vi "Create Folder.vi"(8 "error in":errorcluster, 11 "Source Path":path) -> (0 "error out":errorcluster, 2 "Already Exists":bool, 3 "created path":path)   [LabVIEW 2014, in "Utilities.lvlib"]
uses:
  Utilities.lvlib
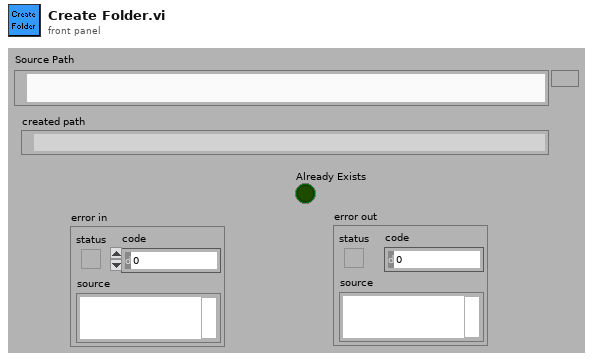
[diagram p1: front panel]
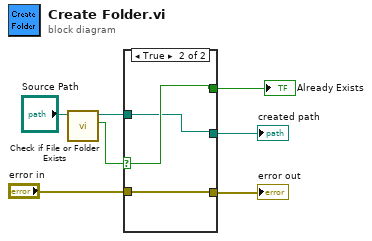
[diagram p0: block diagram]
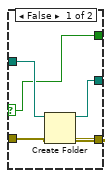
[diagram p2: hidden frame]
diagram:
  n1 = call <vilib>:"Check if File or Folder Exists.vi"("path"="Source Path") -> ("file or folder exists?"=w7:bool, "dup path"=w2:path)  [unwired: 8 in, 1 out]
  n2 = case shown="True" w7 {
    selector: w7 -> [w8 w15]
    tunnel: w2 -> [w11 w13]
    tunnel: "error in" -> [w9 w14]
    tunnel: [w12 w14] -> w4
    tunnel: [w10 w13] -> w3
    tunnel: [w8 w15] -> w1
    frame False {
      n3 = Create Folder(path (use dialog)=w11, error in=w9) -> (created path=w10:path, error out=w12:errorcluster)  [unwired: 1 in, 1 out]
    }
    frame True {
    }
  }
  "error out" <- w4
  "created path" <- w3
  "Already Exists" <- w1
